vi "create default channels.vi"() -> (0 "error out":errorcluster, 1 "names":string[](array[string]), 2 "channels":refnum<class "TBM channel.lvclass">[](array[class]), 3 "module":refnum<class "PID Module configuration.lvclass">, 5 "instance identifier":string)   [LabVIEW 2013, in "Tagbus PID Module tests.lvlib"]
uses:
  Tagbus PID Module tests.lvlib
  <vilib>/NI/Tag Bus Module Framework/channel/TBM channel.lvclass
  module/configuration/PID Module configuration.lvclass
  editor node/PID array element.ctl
  <vilib>/NI/Tag Bus/tag/tag descriptor.lvclass/tag descriptor.ctl
  <vilib>/NI/Configuration Framework/serializable configuration/NISE_CEF_serializable configuration.lvclass
  <vilib>/NI/Tag Bus/tag/tag descriptor.lvclass
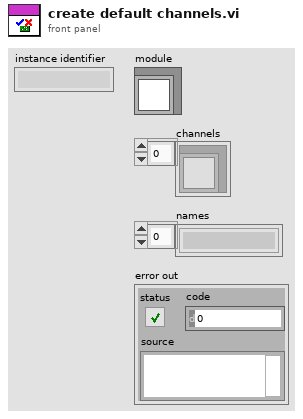
[diagram p1: front panel]
types:
  T1 = typedef "PID Module configuration.lvclass/PID array element.ctl" = cluster{"Loop ID":string, "Tags":cluster{"Setpoint":string, "Process Variable":string, "Output":string}, "Gains":cluster{"P":dbl, "I":dbl, "D":dbl}, "Range":cluster{"High":dbl, "Low":dbl}}
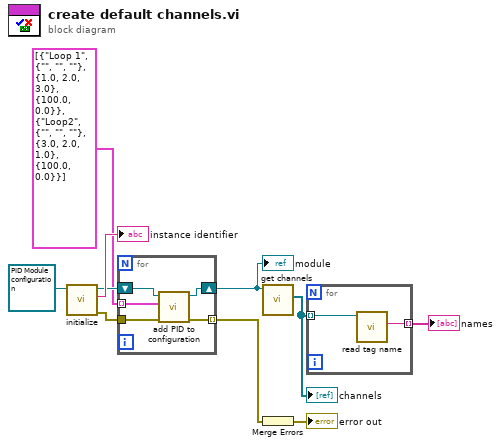
[diagram p0: block diagram]
diagram:
  n1 = call <vilib>:"initialize.vi"("configuration in"=refnum<class "PID Module configuration.lvclass"> refnum ("tag bus configurable plugin module configuration")) -> ("error out"=w8:errorcluster, "identifier"=→"instance identifier":string, "configuration out"=w6:refnum<class "PID Module configuration.lvclass">)  [unwired: 8 in]
  n2 = for {
    tunnel: [w15] -> w10 mode=indexing
    tunnel: w8 -> [w14]
    shift-right: [w13] -> w3
    shift-left: w6 -> [w12]
    tunnel: T1[] [{"Loop ID"="Loop 1", "Tags"={"Setpoint"="", "Process Variable"="", "Output"=""}, "Gains"={"P"=1.0, "I"=2.0, "D"=3.0}, "Range"={"High"=100.0, "Low"=0.0}}, {"Loop ID"="Loop2", "Tags"={"Setpoint"="", "Process Variable"="", "Output"=""}, "Gains"={"P"=3.0, "I"=2.0, "D"=1.0}, "Range"={"High"=100.0, "Low"=0.0}}] ("Array") -> [w11] mode=indexing
    n3 = call "add PID to configuration.vi"("error in"=w14, "PID Element in"=w11, "Tagbus PID Module configuration in"=w12) -> ("error out"=w15:errorcluster, "Tagbus PID Module configuration out"=w13:refnum<class "PID Module configuration.lvclass">)  [unwired: 7 in]
  }
  "module" <- w3
  n4 = call-dynamic "get channels.vi"("module configuration in"=w3) -> ("channels"=w2:refnum<class "TBM channel.lvclass">[])  [unwired: 9 in, 1 out]
  "channels" <- w2
  n5 = Merge Errors(w10) -> (→"error out":errorcluster)
  n6 = for {
    tunnel: w2 -> [w17] mode=indexing
    tunnel: [w16] -> w1 mode=indexing
    n7 = call <vilib>:"read tag name.vi"("system tag in"=w17) -> ("name"=w16:string)  [unwired: 8 in, 2 out]
  }
  "names" <- w1
